vi "Add Modules to Slot List (ChGrp).vi"(8 "error in (no error)":errorcluster, 10 "ChanGrp.lvclass":refnum<class "ChanGrp.lvclass">, 11 "SlotMod List in":string[](array[string])) -> (0 "error out":errorcluster, 3 "SlotMod List out":string[](array[string]))   [LabVIEW 2018, in "Configuration Grandmaster.lvlib" / "ChanGrp.lvclass"]
uses:
  ChanGrp.lvclass
  ChanGrp.lvclass/ChanGrp.ctl
  Measurements/Class Channel/Read ChanName.vi
  Measurements/Class Channel/Read Device.vi
  Measurements/Class Channel/Channel.lvclass
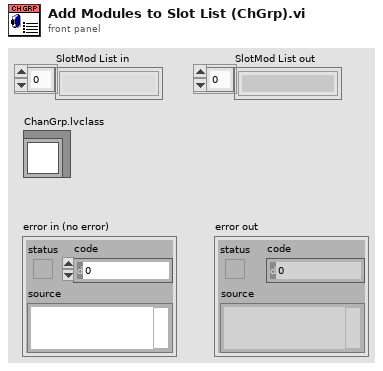
[diagram p1: front panel]
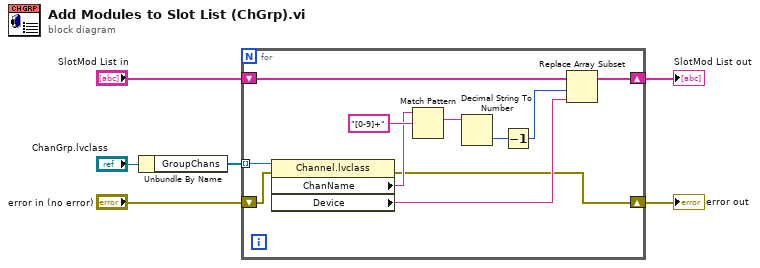
[diagram p0: block diagram]
diagram:
  n1 = Unbundle By Name("ChanGrp.lvclass") -> ("GroupChans"=w3:refnum<class "Channel.lvclass">[])
  n2 = for {
    shift-right: [w12] -> w6
    shift-left: "SlotMod List in" -> [w14]
    tunnel: w3 -> [w9] mode=indexing
    shift-right: [w7] -> w1
    shift-left: "error in (no error)" -> [w8]
    n3 = property class="Channel.lvclass"(reference=w9, error in=w8) -> (error out=w7:errorcluster, "ChanName"=w11:string, "Device"=w10:string)  [unwired: 1 out]
    n4 = Match Pattern(string=w11, regular expression="[0-9]+") -> (match substring=w17:string)  [unwired: 1 in, 3 out]
    n5 = Decimal String To Number(string=w17) -> (number=w15:i32)  [unwired: 2 in, 1 out]
    n6 = Decrement(x=w15) -> (x-1=w13:i32)
    n7 = Replace Array Subset(array=w14, new element=w10, index=w13) -> (w12:string[])
  }
  "SlotMod List out" <- w6
  "error out" <- w1
